vi "Submit all intermediate structures script.vi"() -> ()   [LabVIEW 2010]
uses:
  <vilib>/Utility/file.llb/Write To Spreadsheet File (string).vi
panel:
  in  "# Frames":i32=10
  in  "Directory 1":path=path "D:/Ab-initio/VASP Calcs/2D_Grain Boundaries/Batch51_20131230/Bulk_111_supercell"
  in  "New DIrectory":path=path "D:/Ab-initio/VASP Calcs/2D_Grain Boundaries/Batch51_20131230"
  in  "Directory 2":path=path "D:/Ab-initio/VASP Calcs/2D_Grain Boundaries/Batch51_20131230/A3B3"
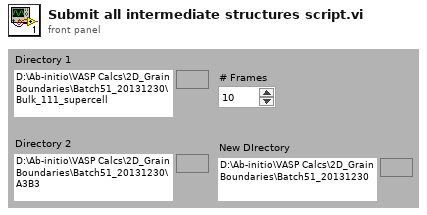
[diagram p1: front panel]
types:
  T1 = cluster{"Structure Name":string, "Lattice vector a":dbl[], "Lattice vector b":dbl[], "Lattice vector c":dbl[], "Atoms Array":cluster{"Atom Name":string, "Positions (Direct)":dbl[][], "Positions (Cartesian)":dbl[][]}[], "# of atoms":i32}
  T2 = cluster{"Structure Name":string, "Lattice vector a":dbl[], "Lattice vector b":dbl[], "Lattice vector c":dbl[], "Atoms Array":cluster{"Atom Name":string, "Positions (Direct)":dbl[][], "Positions (Cartesian)":dbl[][]}[], "# of atoms":i32}[]
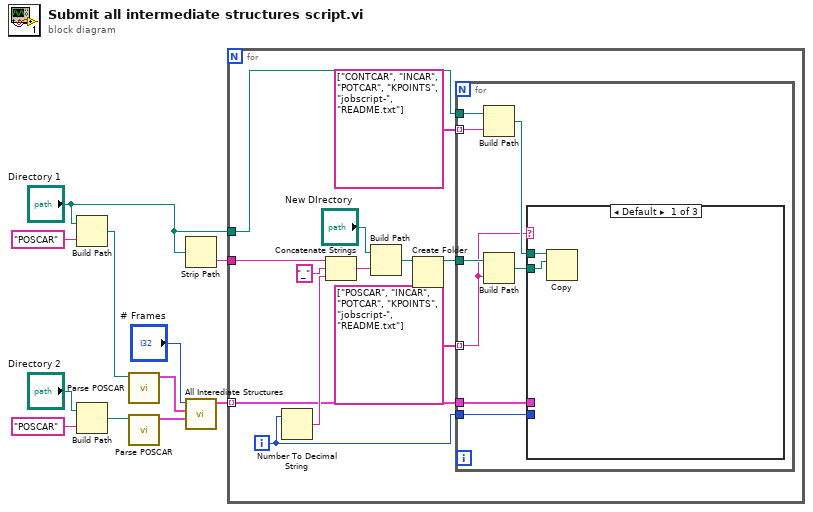
[diagram p0: block diagram]
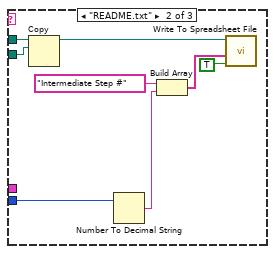
[diagram p2: hidden frame]
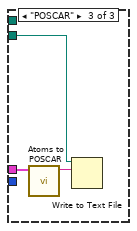
[diagram p3: hidden frame]
diagram:
  n1 = Build Path(base path="Directory 1", name or relative path="POSCAR") -> (appended path=w2:path)
  n2 = Build Path(base path="Directory 2", name or relative path="POSCAR") -> (appended path=w6:path)
  n3 = call "Parse POSCAR.vi"("POSCAR File"=w2) -> ("Structure"=w11:T1)  [unwired: 7 in, 3 out]
  n4 = call "Parse POSCAR.vi"("POSCAR File"=w6) -> ("Structure"=w10:T1)  [unwired: 7 in, 3 out]
  n5 = Strip Path(path="Directory 1") -> (name=w3:string)  [unwired: 1 out]
  n6 = call "All Interediate Structures.vi"("Second Structure"=w10, "First Structure"=w11, "# Frames"="# Frames") -> ("Array of Structures"=w5:T2)  [unwired: 8 in]
  n7 = for {
    tunnel: w5 -> [w14] mode=indexing
    tunnel: w3 -> [w16]
    tunnel: "Directory 1" -> [w12]
    i -> [w15]
    n8 = Number To Decimal String(number=w15) -> (decimal integer string=w17:string)  [unwired: 1 in]
    n9 = Concatenate Strings(w16, "_" ("string"), w17) -> (w18:string)
    n10 = Build Path(base path="New DIrectory", name or relative path=w18) -> (appended path=w22:path)
    n11 = Create Folder(path (use dialog)=w22) -> (created path=w21:path)  [unwired: 2 in, 2 out]
    n12 = for {
      tunnel: w12 -> [w31]
      tunnel: w21 -> [w28]
      tunnel: string[] ["CONTCAR", "INCAR", "POTCAR", "KPOINTS", "jobscript-", "README.txt"] -> [w30] mode=indexing
      tunnel: string[] ["POSCAR", "INCAR", "POTCAR", "KPOINTS", "jobscript-", "README.txt"] -> [w26] mode=indexing
      tunnel: w15 -> [w25]
      tunnel: w14 -> [w24]
      n13 = Build Path(base path=w31, name or relative path=w30) -> (appended path=w29:path)
      n14 = Build Path(base path=w28, name or relative path=w26) -> (appended path=w27:path)
      n15 = case shown="Default" w26 {
        tunnel: w29 -> [w33 w40 _]
        tunnel: w27 -> [w32 w41 w42]
        tunnel: w25 -> [_ w37 _]
        tunnel: w24 -> [_ _ w44]
        frame Default {
          n16 = Copy(10:w32, 11:w33) -> ()  [unwired: 3 in, 3 out]
        }
        frame "README.txt" {
          n17 = Copy(10:w41, 11:w40) -> (3:w34:path)  [unwired: 3 in, 2 out]
          n18 = Number To Decimal String(number=w37) -> (decimal integer string=w36:string)  [unwired: 1 in]
          n19 = Build Array("Intermediate Step #", w36) -> (w35:string[])
          n20 = call-poly <vilib>:"Write To Spreadsheet File.vi"("append to file? (new file:F)"=TRUE, "1D data"=w35, "file path (dialog if empty)"=w34) -> ()  [unwired: 5 in, 1 out]
        }
        frame "POSCAR" {
          n21 = call "Atoms to POSCAR.vi"("Atomic Structure"=w44) -> ("POSCAR File"=w43:string)  [unwired: 10 in]
          n22 = Write to Text File(file (use dialog)=w42, text=w43) -> ()  [unwired: 2 in, 3 out]
        }
      }
    }
  }
